vi "SendSMTP_Email_2.vi"(4 "Send as attachment":bool, 5 "message":string="This email was sent to you via labview SMTP email.!", 6 "message (attachment)":string, 7 "subject ([No Subject])":string="<Automatic Email> Do not respond!", 8 "error in (no error)":errorcluster, 10 "file path":path[](array[path]), 11 "Recipient Email Address":string) -> (0 "error out":errorcluster)   [LabVIEW 2018]
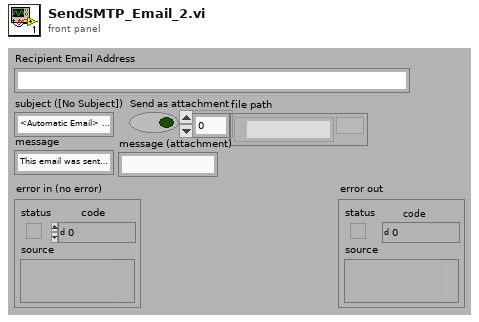
[diagram p1: front panel]
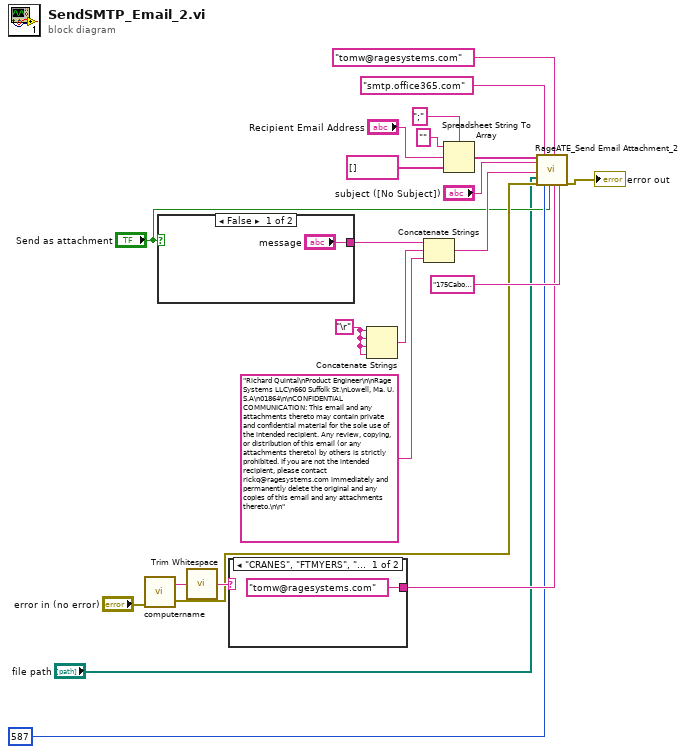
[diagram p0: block diagram]
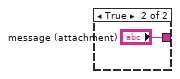
[diagram p2: hidden frame]
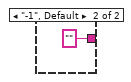
[diagram p3: hidden frame]
diagram:
  w17 = "\r"
  n1 = call "computername.vi"("error in (no error)"="error in (no error)") -> ("error out"=w4:errorcluster, "String/Binary data"=w14:string)  [unwired: 3 in]
  n2 = case shown="False" "Send as attachment" {
    tunnel: ["message" "message (attachment)"] -> w19
    frame False {
    }
    frame True {
    }
  }
  n3 = call <vilib>:"Trim Whitespace.vi"("string"=w14) -> ("trimmed string"=w13:string)  [unwired: 1 in]
  n4 = case shown="\"CRANES\", \"FTMYERS\", \"HAMPTON\"" w13 {
    tunnel: ["tomw@ragesystems.com" ("Mail Server 2") "" ("Mail Server 2")] -> w6
    frame "CRANES", "FTMYERS", "HAMPTON" {
    }
    frame "-1", Default {
    }
  }
  n5 = Concatenate Strings(w17, w17, w17, w17) -> (w18:string)
  n6 = Concatenate Strings(w19, w18, "Richard Quintal\nProduct Engineer\n\nRage Systems LLC\n660 Suffolk St.\nLowell, Ma. U.S.A\n01864\n\nCONFIDENTIAL COMMUNICATION: This email and any attachments thereto may contain private and confidential material for the sole use of the intended recipient. Any review, copying, or distribution of this email (or any attachments thereto) by others is strictly prohibited. If you are not the intended recipient, please contact rickq@ragesystems.com immediately and permanently delete the original and any copies of this email and any attachments thereto.\n\n") -> (w10:string)
  n7 = Spreadsheet String To Array(delimiter (Tab)=";", format string="", spreadsheet string="Recipient Email Address", array type (2D Dbl)=string[] []) -> (array=w12:string[])
  n8 = call "RageATE_Send Email Attachment_2.vi"("To: (email@site.com)"=w12, "Subject:"="subject ([No Subject])", "Body:"=w10, "Attachment Path"="file path", "error in (no error)"=w4, "SMTP Outgoing Mail Server"="smtp.office365.com", "Port"=587, "Send Attachment(t)"="Send as attachment", "From: (email@site.com)"="tomw@ragesystems.com" ("Email Account ID"), "Email Account ID"=w6, "Email Account Password"="175CabotSt!") -> ("error out"=→"error out":errorcluster)  [unwired: 8 in]
